vi "createInstance.vi"(8 "error in (no error)":errorcluster, 9 "salTypedefPath":path=path "C:/LSSTSW/SAL_LabVIEW_Interface/SALTypedefs/Control 2.ctl", 10 "instanceDirectory":path, 11 "PolymorphicInstance in":refnum<class "PolymorphicInstance.lvclass">) -> (0 "error out":errorcluster, 3 "PolymorphicInstance out":refnum<class "PolymorphicInstance.lvclass">)   [LabVIEW 2012, in "PolymorphicInstance.lvclass"]
uses:
  PolymorphicInstance.lvclass
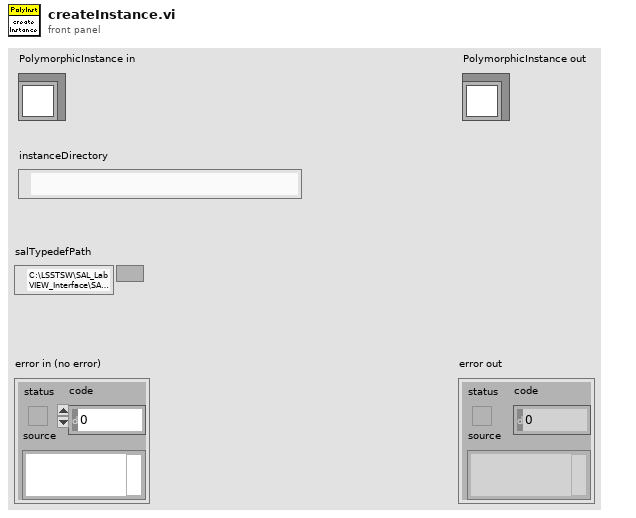
[diagram p1: front panel]
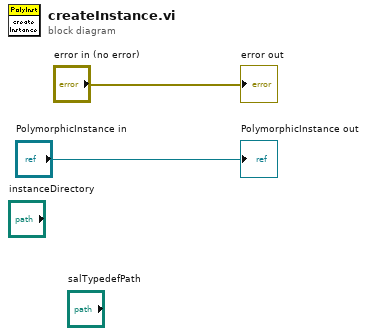
[diagram p0: block diagram]
diagram:
  "error out" <- "error in (no error)"
  "PolymorphicInstance out" <- "PolymorphicInstance in"
